vi "Get Item Real Name from Full Name.vi"(11 "Full name with lib/class prefix":string) -> (3 "real short name":string)   [LabVIEW 2014]
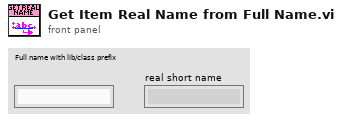
[diagram p1: front panel]
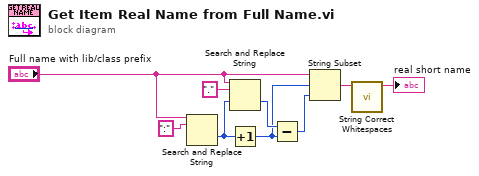
[diagram p0: block diagram]
diagram:
  n1 = Search and Replace String(input string="Full name with lib/class prefix", search string=":" ("regular expression")) -> (offset past replacement=w4:i32)  [unwired: 6 in, 3 out]
  n2 = Search and Replace String(input string="Full name with lib/class prefix", search string="." ("regular expression"), offset=w4) -> (offset past replacement=w2:i32)  [unwired: 5 in, 3 out]
  n3 = Increment(x=w4) -> (x+1=w1:i32)
  n4 = Subtract(x=w2, y=w1) -> (x-y=w3:i32)
  n5 = String Subset(string="Full name with lib/class prefix", offset (0)=w1, length (rest)=w3) -> (substring=w8:string)
  n6 = call "String Correct Whitespaces.vi"("String in"=w8) -> ("String out"=→"real short name":string)  [unwired: 10 in]
